vi "未命名 6.vi"() -> ()   [LabVIEW 2020]
panel:
  out "变体":variant
  out "全打开":T1
  out "电压检测":T2
  # "320±3"
  # "≤1"
  # "≤1"
  # "≤1"
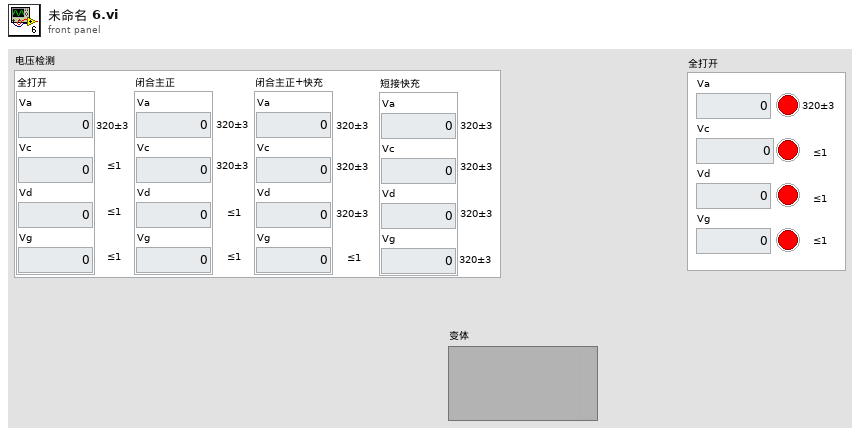
[diagram p1: front panel]
types:
  T1 = cluster{"Va":u32, "Vc":u32, "Vd":u32, "Vg":u32, bool, bool, bool, bool}
  T2 = typedef "电压检测.ctl" = cluster{"全打开":cluster{"Va":u32, "Vc":u32, "Vd":u32, "Vg":u32}, "闭合主正":cluster{"Va":u32, "Vc":u32, "Vd":u32, "Vg":u32}, "闭合主正+快充":cluster{"Va":u32, "Vc":u32, "Vd":u32, "Vg":u32}, "短接快充":cluster{"Va":u32, "Vc":u32, "Vd":u32, "Vg":u32}}
  T3 = enum8{"Enabled", "Disabled", "Disabled and Grayed Out"}
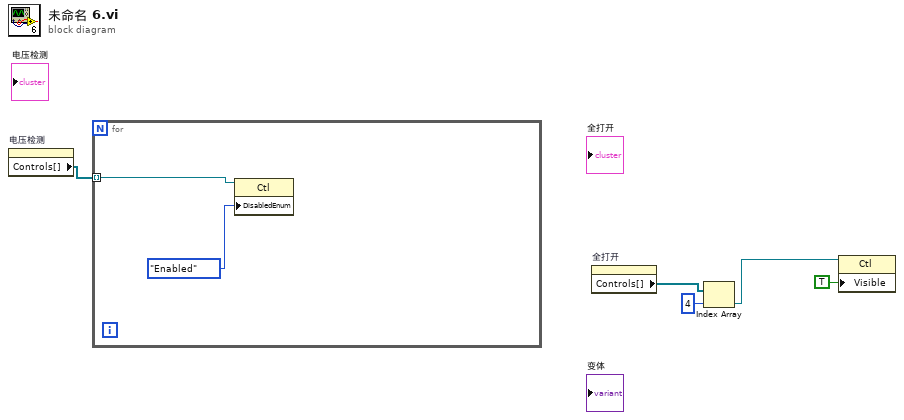
[diagram p0: block diagram]
diagram:
  n1 = property on="电压检测" class="Clust (严格)"() -> ("Controls[]"=w5:refnum<vi>[])  [unwired: 2 in, 2 out]
  n2 = for {
    tunnel: w5 -> [w7] mode=indexing
    n3 = property class="Ctl"(reference=w7, "DisabledEnum"=T3."Enabled" ("禁用")) -> ()  [unwired: 1 in, 2 out]
  }
  n4 = property on="全打开" class="Clust (严格)"() -> ("Controls[]"=w4:refnum<vi>[])  [unwired: 2 in, 2 out]
  n5 = Index Array(array=w4, index=4 ("索引")) -> (element=w1:refnum<vi>)
  n6 = property class="Ctl"(reference=w1, "Visible"=TRUE ("可见")) -> ()  [unwired: 1 in, 2 out]
